vi "Motor_GetAngleSpeed(nofilter).vi"(6 "initialize":bool, 8 "dt":dbl=1.0 format="%0.2f", 9 "Initial Condition":dbl[](array[numeric]) format="%0.2f", 11 "Angles":dbl[](array[numeric]) format="%0.2f") -> (3 "AngularSpeed":dbl[](array[numeric]))   [LabVIEW 2015, in "MotorControl.lvclass"]
uses:
  MotorControl.lvclass
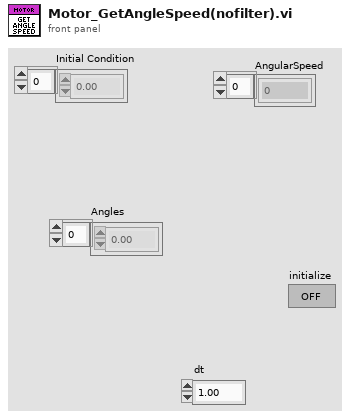
[diagram p1: front panel]
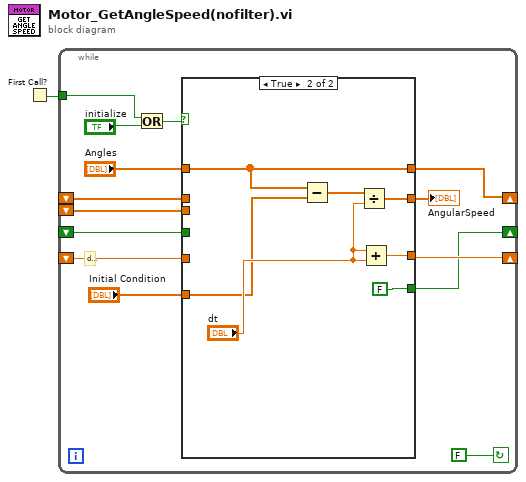
[diagram p0: block diagram]
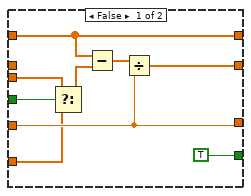
[diagram p2: hidden frame]
diagram:
  n1 = First Call?() -> (First Call?: T/F=w1:bool)
  n2 = while {
    shift-left: _ -> [w6]
    shift-right: [w7] -> _
    shift-left: _ -> [w10]
    shift-right: [w11] -> _
    tunnel: w1 -> [w14]
    shift-left: _ -> [w9]
    shift-left: _ -> [w5]
    shift-right: [w8] -> _
    stop <- FALSE continue-if-true
    # "dt"
    n3 = Or(x=w14, y="initialize") -> (x .or. y?=w12:bool)
    n4 = case shown="True" w12 {
      tunnel: [w22 w27] -> w11
      tunnel: "Angles" -> [w23 w29]
      tunnel: [w24 w30] -> w2
      tunnel: w10 -> [w22 _]
      tunnel: w9 -> [w18 _]
      tunnel: [w23 w29] -> w8
      tunnel: [TRUE FALSE] -> w7
      tunnel: w6 -> [w19 _]
      tunnel: w5 -> [_ _]
      tunnel: "Initial Condition" -> [w17 w25]
      frame False {
        n5 = Select(t=w18, s=w19, f=w17) -> (s? t:f=w16:dbl[])
        n6 = Subtract(x=w23, y=w16) -> (x-y=w20:dbl[])
        n7 = Divide(x=w20, y=w22) -> (x/y=w24:dbl[])
      }
      frame True {
        n8 = Subtract(x=w29, y=w25) -> (x-y=w31:dbl[])
        n9 = Divide(x=w31, y="dt") -> (x/y=w30:dbl[])
        n10 = Add(x="dt", y="dt") -> (x+y=w27:dbl)
      }
    }
    "AngularSpeed" <- w2
  }
